vi "Tension à température.vi"() -> ()   [LabVIEW 2018]
panel:
  out "Température":dbl(slide) scale=0.0..100.0
  in  "Tension":dbl(slide) scale=0.0..10.0
  # "Sous-VI qui calcule la conversion de la tension en température"
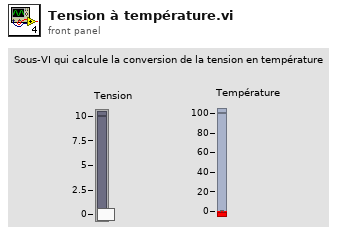
[diagram p1: front panel]
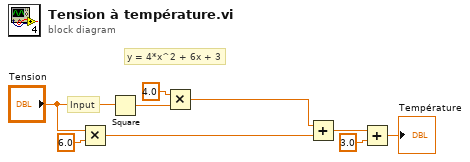
[diagram p0: block diagram]
diagram:
  # "y = 4*x^2 + 6x + 3"
  # "Input"
  n1 = Multiply(x="Tension", y=6.0) -> (x*y=w5:dbl)
  n2 = Square(x="Tension") -> (x^2=w8:dbl)
  n3 = Multiply(x=4.0, y=w8) -> (x*y=w7:dbl)
  n4 = Add(x=w7, y=w5) -> (x+y=w4:dbl)
  n5 = Add(x=w4, y=3.0) -> (x+y=→"Température":dbl)
